vi "KE_Acquire.vi"(6 "KeepOn?":bool=TRUE, 7 "Type":u16(ring) items=["First", "Second", "Init"], 8 "error in (no error)":errorcluster, 11 "Instruments in":refnum<class "Instruments.lvclass">) -> (0 "error out":errorcluster, 3 "Instruments out":refnum<class "Instruments.lvclass">, 5 "Voltage":dbl)   [LabVIEW 2012, in "Instruments.lvclass"]
uses:
  Instruments.lvclass
  Instruments.lvclass/Instruments.ctl
  Instruments/Drivers/ke236/KE236.LLB/Keith 236 Operate/Standby.vi
panel:
  in  "integration time (medium:1)":u16(ring)=1 items=["fast perod", "medium period", "line cycle period @ 50Hz", "line cycle period @ 60Hz"]
  out "device dependent errors":string
  out "?":T1(array[cluster])
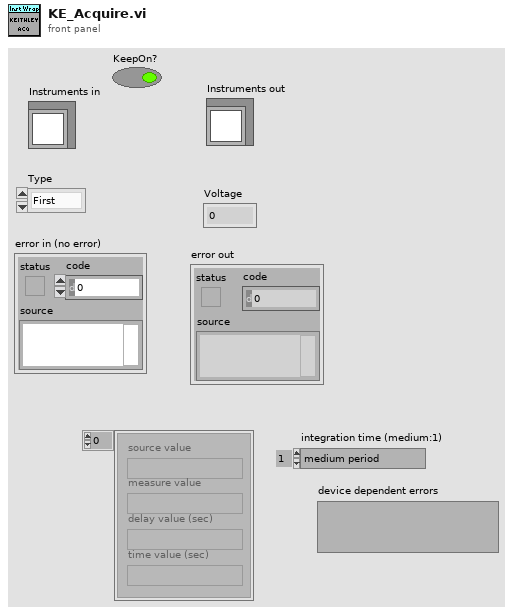
[diagram p1: front panel]
types:
  T1 = cluster{"source value":string, "measure value":string, "delay value (sec)":string, "time value (sec)":string}[]
  T2 = typedef "SMUParam.ctl" = cluster{"Start Current,mA":dbl, "Stop Current,mA":dbl, "Voltage Compliance,V":dbl, "GPIB":string, "VISA resource name":refnum<visa-resource-name>}
  T3 = cluster{"error":bool, "code":i32, "source":string}
  T4 = cluster{"source value":string, "measure value":string, "delay value (sec)":string, "time value (sec)":string}
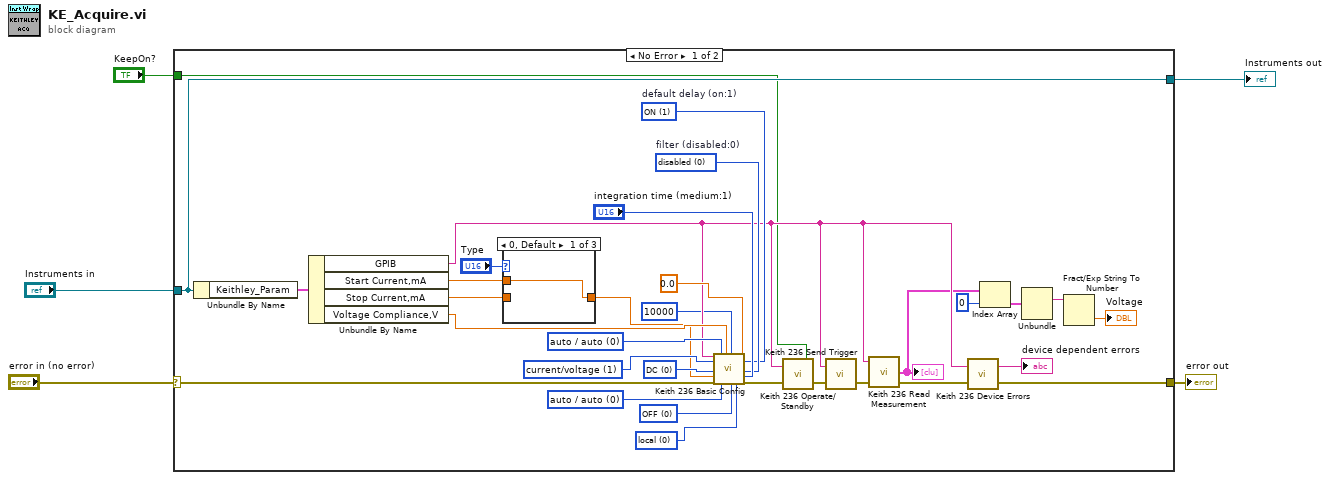
[diagram p0: block diagram]
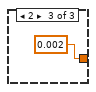
[diagram p3: hidden frame]
diagram:
  n1 = case shown="No Error" "error in (no error)" {
    selector: "error in (no error)" -> [w19 w42]
    tunnel: [w21 w42] -> w4
    tunnel: [w20 w41] -> w2
    tunnel: "Instruments in" -> [w20 w41]
    tunnel: "KeepOn?" -> [w15 _]
    frame No Error {
      w28 = u16 1 items=["OFF", "ON"]  # default delay (on:1)
      w29 = u16 0 items=["disabled", "2 readings", "4 readings", "8 readings", "16 readings", "32 readings"]  # filter (disabled:0)
      w32 = u16 0 items=["local", "remote"] ("sense (local:0)")
      w33 = u16 0 items=["OFF", "ON"] ("suppression (off:0)")
      w34 = u16 0 items=["auto / auto", "1 nA / 1.1 V", "10 nA / 11 V", "100 nA / 110 V", "0.001 mA / 110 V", "0.01 mA / 110 V", "0.1 mA / 110 V", "1 mA / 110 V", "10 mA / 110 V", "100 mA / 110 V"] ("compliance/\nmeasurement range (auto:0)")
      w35 = u16 0 items=["DC", "sweep"] ("function (DC:0)")
      w36 = u16 1 items=["voltage/current", "current/voltage"] ("source/measure (V/I:0)")
      w37 = u16 0 items=["auto / auto", "1 nA / 1.1 V", "10 nA / 11 V", "100 nA / 110 V", "0.001 mA / 110 V", "0.01 mA / 110 V", "0.1 mA / 110 V", "1 mA / 110 V", "10 mA / 110 V", "100 mA / 110 V"] ("source range\nI source / V source (auto:0)")
      n2 = Unbundle By Name(w20) -> ("Keithley_Param"=w18:T2)
      n3 = Unbundle By Name(w18) -> ("GPIB"=w26:string, "Start Current,mA"=w24:dbl, "Stop Current,mA"=w23:dbl, "Voltage Compliance,V"=w27:dbl)
      n4 = case shown="0, Default" "Type" {
        tunnel: w24 -> [w38 _ _]
        tunnel: w23 -> [_ w39 _]
        tunnel: [w38 w39 0.002 ("Stop Current,mA")] -> w22
        frame 0, Default {
        }
        frame 1 {
        }
        frame 2 {
        }
      }
      n5 = call "Keith 236 Basic Config.vi"("GPIB address"=w26, "source/measure (V/I:0)"=w36, "function (DC:0)"=w35, "source level"=w22, "error in"=w19, "source range\nI source / V source (auto:0)"=w37, "compliance/\nmeasurement range (auto:0)"=w34, "voltage \ncompliance level"=w27, "timeout ms"=u32 10000, "suppression (off:0)"=w33, "sense (local:0)"=w32, "DC delay (sec)"=0.0, "default delay (on:1)"=w28, "filter (disabled:0)"=w29, "integration time (medium:1)"="integration time (medium:1)") -> ("error out"=w16:T3)  [unwired: 4 in]
      n6 = call "Keith 236 Operate/Standby.vi"("source"=w15, "error in"=w16, "GPIB address"=w26) -> ("error out"=w6:T3)
      n7 = call "Keith 236 Send Trigger.vi"("GPIB address"=w26, "error in"=w6) -> ("error out"=w13:T3)
      n8 = call "Keith 236 Read Measurement.vi"("error in"=w13, "GPIB address"=w26) -> ("error out"=w14:T3, "display"=w11:T1)  [unwired: 2 out]
      "?" <- w11
      n9 = call "Keith 236 Device Errors.vi"("error in"=w14, "GPIB address"=w26) -> ("error out"=w21:T3, "device dependent errors"=→"device dependent errors":string)
      n10 = Index Array(array=w11, index=0) -> (element=w9:T4)
      n11 = Unbundle(w9) -> ("measure value"=w8:string)  [unwired: 3 out]
      n12 = Fract/Exp String To Number(string=w8) -> (number=→"Voltage":dbl)  [unwired: 3 in, 1 out]
    }
    frame Error {
    }
  }
  "error out" <- w4
  "Instruments out" <- w2
